vi "Add New Line.vi"(8 "error in":errorcluster, 11 "objects":T1) -> (0 "error out":errorcluster, 1 "success":bool)   [LabVIEW 2013, in "OPC UA editor node.lvclass"]
doc: "This VI is called to add new elements to the configuration. \nIt creates a new default line and the opens the dialog to edit its properties. \nFinally it adds it to the configuration."
uses:
  OPC UA editor node.lvclass
  <vilib>/NI/DCAF Table API/Table Manager/object ref.ctl
  <vilib>/NI/DCAF/Tag Editor Core/Configuration Editor/Classes/Engine Parent/Engine Parent Editor Node.lvclass
  <vilib>/NI/DCAF/Tag Editor Core/Configuration Editor/Classes/Module editor node/module editor node.lvclass
  <vilib>/NI/DCAF Table API/Table Manager/Table Manager.lvclass
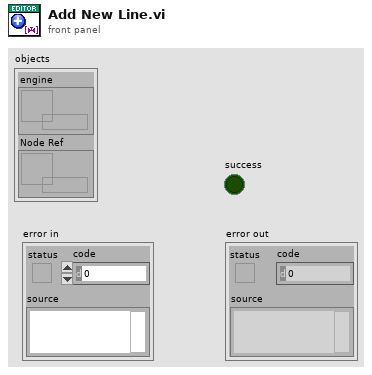
[diagram p1: front panel]
types:
  T1 = typedef "Table Manager.lvlib/Table Manager.lvclass/object ref.ctl" = cluster{"engine":refnum<data-value>, "Node Ref":refnum<data-value>}
  T2 = typedef "OPC UA configuration.lvclass/Line.ctl" = cluster{"channel":refnum<class "TBM channel.lvclass">, "Node Path":string, "OPC UA Data Type":enum16{"Bool", "SByte", "Byte", "Int16", "UInt16", "Int32", "UInt32", "Int64", "UInt64", "Float", "Double", "String", "DateTime", "ByteString", "Bool Array", "SByte Array", "Byte Array", "Int16 Array", "UInt16 Array", "Int32 Array", "UInt32 Array", "Int64 Array", "UInt64 Array", "Float Array", "Double Array", "String Array", "DateTime Array", "ByteString Array"}}
  T3 = typedef "OPC UA editor node.lvclass/Mappings.ctl" = cluster{"Line":T2, "Maps":T4[]}
  T4 = typedef "OPC UA editor node.lvclass/Map.ctl" = cluster{"channel":refnum<class "TBM channel.lvclass">, "tag name":string}
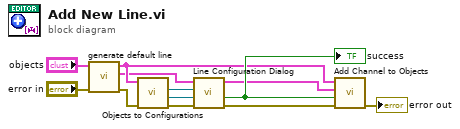
[diagram p0: block diagram]
diagram:
  n1 = call "generate default line.vi"("error in"="error in", "objects in"="objects") -> ("error out"=w3:errorcluster, "Line"=w4:T2, "objects out"=w7:T1)  [unwired: 7 in]
  n2 = call "Objects to Configurations.vi"("error in (no error)"=w3, "Objects in"=w7) -> ("error out"=w6:errorcluster, "engine configuration out"=w1:refnum<class "engine configuration.lvclass">, "tag bus configurable plugin module configuration"=w2:refnum<class "OPC UA configuration.lvclass">)  [unwired: 7 in]
  n3 = call "Line Configuration Dialog.vi"("error in"=w6, "engine configuration in"=w1, "tag bus configurable plugin module configuration"=w2, "Line"=w4) -> ("error out"=w10:errorcluster, "success"=w8:bool, "Mappings out"=w5:T3)  [unwired: 4 in, 1 out]
  "success" <- w8
  n4 = call "Add Channel to Objects.vi"("error in"=w10, "success"=w8, "line item in"=w5, "Objects in"=w7) -> ("error out"=→"error out":errorcluster)  [unwired: 7 in]
